vi "BatchFGV.vi"(7 "FGV Ops":T3, 8 "error in (no error)":errorcluster, 11 "SetCurrentBatch":T1) -> (0 "error out":errorcluster, 3 "GetCurrentBatch":T1)   [LabVIEW 2024]
uses:
  CTRLS/FVG Ops.ctl
  CTRLS/SetCurrentBatch inputs.ctl
  CTRLS/Recipe info.ctl
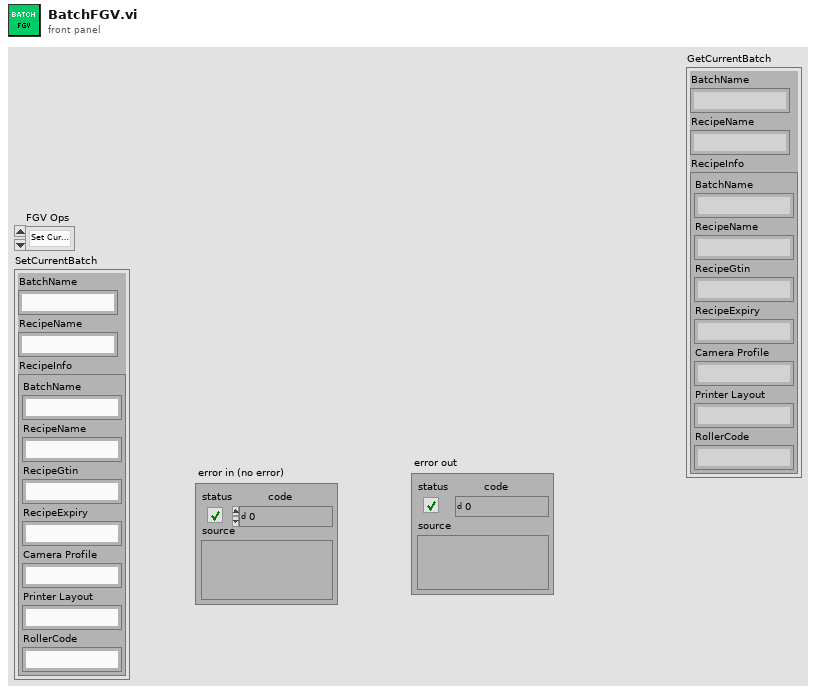
[diagram p1: front panel]
types:
  T1 = typedef "SetCurrentBatch inputs.ctl" = cluster{"BatchName":string, "RecipeName":string, "RecipeInfo":T2}
  T2 = typedef "Recipe info.ctl" = cluster{"BatchName":string, "RecipeName":string, "RecipeGtin":string, "RecipeExpiry":string, "Camera Profile":string, "Printer Layout":string, "RollerCode":string}
  T3 = typedef "FVG Ops.ctl" = enum16{"Set Current Batch", "Get Current Batch", "Set Current Recipe", "Get Current Recipe"}
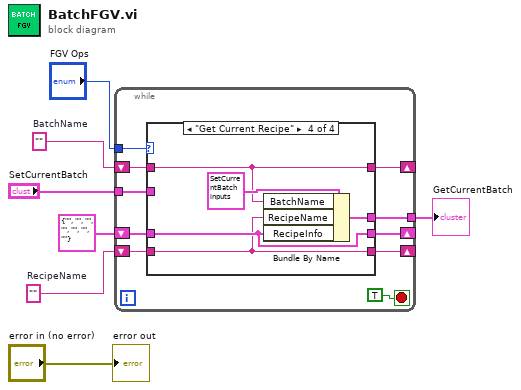
[diagram p0: block diagram]
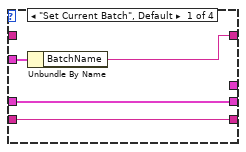
[diagram p2: hidden frame]
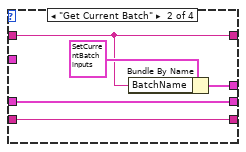
[diagram p3: hidden frame]
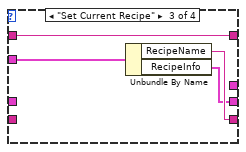
[diagram p4: hidden frame]
diagram:
  w4 = ""  # BatchName
  w5 = ""  # RecipeName
  n1 = while {
    tunnel: "FGV Ops" -> [w16]
    shift-right: [w14] -> _
    shift-left: w4 -> [w15]
    shift-right: [w12] -> _
    shift-left: w5 -> [w11]
    tunnel: "SetCurrentBatch" -> [w13]
    shift-right: [w10] -> _
    shift-left: T2 {"BatchName"="", "RecipeName"="", "RecipeGtin"="", "RecipeExpiry"="", "Camera Profile"="", "Printer Layout"="", "RollerCode"=""} ("RecipeInfo") -> [w9]
    tunnel: [w8] -> w2
    stop <- TRUE stop-if-true
    n2 = case shown="\"Get Current Recipe\"" w16 {
      tunnel: w15 -> [_ w25 w30 w33]
      tunnel: [w21 w25 w30 w33] -> w14
      tunnel: w13 -> [w20 _ w29 _]
      tunnel: [w19 w24 w28 w32] -> w12
      tunnel: w11 -> [w19 w24 _ w32]
      tunnel: [w18 w23 w27 w34] -> w10
      tunnel: w9 -> [w18 w23 _ w34]
      tunnel: [_ w22 _ w31] -> w8
      frame "Set Current Batch", Default {
        n3 = Unbundle By Name(w20) -> ("BatchName"=w21:string)
      }
      frame "Get Current Batch" {
        n4 = Bundle By Name(cluster=T1 {"BatchName"="batch1", "RecipeName"="asd", "RecipeInfo"={"BatchName"="", "RecipeName"="", "RecipeGtin"="", "RecipeExpiry"="", "Camera Profile"="", "Printer Layout"="", "RollerCode"=""}} ("GetCurrentBatch"), "BatchName"=w25) -> (w22:T1)
      }
      frame "Set Current Recipe" {
        n5 = Unbundle By Name(w29) -> ("RecipeName"=w28:string, "RecipeInfo"=w27:T2)
      }
      frame "Get Current Recipe" {
        n6 = Bundle By Name(cluster=T1 {"BatchName"="batch1", "RecipeName"="asd", "RecipeInfo"={"BatchName"="", "RecipeName"="", "RecipeGtin"="", "RecipeExpiry"="", "Camera Profile"="", "Printer Layout"="", "RollerCode"=""}} ("GetCurrentBatch"), "BatchName"=w33, "RecipeName"=w32, "RecipeInfo"=w34) -> (w31:T1)
      }
    }
  }
  "GetCurrentBatch" <- w2
  "error out" <- "error in (no error)"
